vi "GetAppearance.vi"(8 "error in (no error)":errorcluster, 11 "Column in":refnum<class "Column.lvclass">) -> (0 "error out":errorcluster, 2 "Column Appearance":T1={"Column Name"="", "Width"=30, "Bkgd"=[16448250], "Text"=[0]}, 3 "Column out":refnum<class "Column.lvclass">)   [LabVIEW 2013, in "Column.lvclass"]
uses:
  Column.lvclass
  TypeDefs/ColumnAppearCluster.ctl
  Column.lvclass/Column.ctl
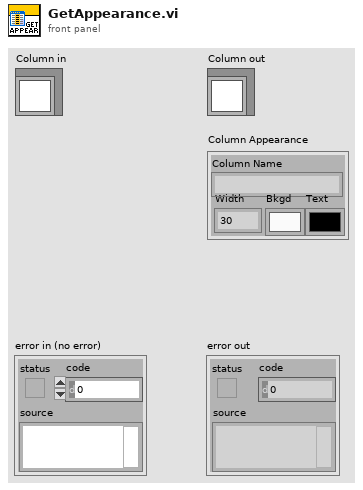
[diagram p1: front panel]
types:
  T1 = typedef "ColumnAppearCluster.ctl" = cluster{"Column Name":string, "Width":u32, "Bkgd":u32[], "Text":u32[]}
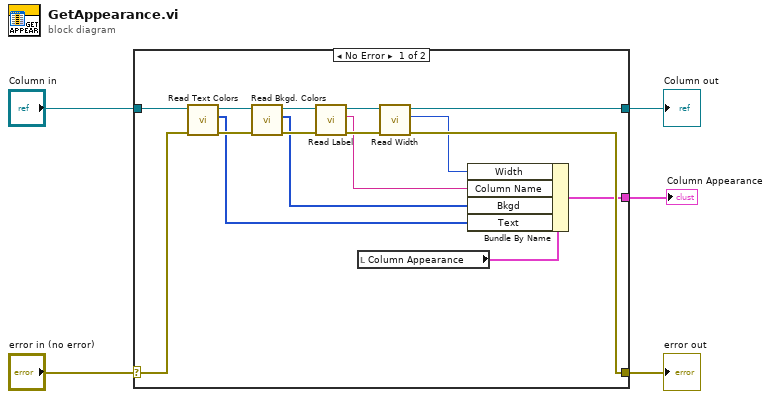
[diagram p0: block diagram]
diagram:
  n1 = case shown="No Error" "error in (no error)" {
    selector: "error in (no error)" -> [w12 w23]
    tunnel: [w11 w23] -> w4
    tunnel: [w16 w22] -> w2
    tunnel: "Column in" -> [w17 w22]
    tunnel: [w6 _] -> w1
    frame No Error {
      n2 = call "Read Text Colors.vi"("error in (no error)"=w12, "Column in"=w17) -> ("error out"=w15:errorcluster, "Text Colors"=w7:u32[], "Column out"=w20:refnum<class "Column.lvclass">)  [unwired: 7 in]
      n3 = call "Read Bkgd. Colors.vi"("error in (no error)"=w15, "Column in"=w20) -> ("error out"=w14:errorcluster, "Bkgd. Colors"=w8:u32[], "Column out"=w19:refnum<class "Column.lvclass">)  [unwired: 7 in]
      n4 = call "Read Label.vi"("error in (no error)"=w14, "Column in"=w19) -> ("error out"=w13:errorcluster, "Label"=w9:string, "Column out"=w18:refnum<class "Column.lvclass">)  [unwired: 7 in]
      n5 = local read "Column Appearance"() -> (w21:T1)
      n6 = call "Read Width.vi"("error in (no error)"=w13, "Column in"=w18) -> ("error out"=w11:errorcluster, "Width"=w10:u32, "Column out"=w16:refnum<class "Column.lvclass">)  [unwired: 7 in]
      n7 = Bundle By Name(cluster=w21, "Width"=w10, "Column Name"=w9, "Bkgd"=w8, "Text"=w7) -> (w6:T1)
    }
    frame Error {
    }
  }
  "error out" <- w4
  "Column out" <- w2
  "Column Appearance" <- w1
